vi "Update_FrontPanel.vi"(8 "End":timestamp, 9 "Start":timestamp, 11 "XYGraph in":refnum<vi>) -> ()   [LabVIEW 2020]
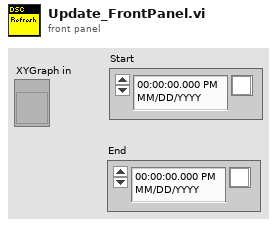
[diagram p1: front panel]
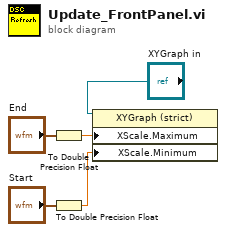
[diagram p0: block diagram]
diagram:
  n1 = To Double Precision Float(number="End") -> (double precision float=w3:dbl)
  n2 = To Double Precision Float(number="Start") -> (double precision float=w1:dbl)
  n3 = property on="Property Node" class="XYGraph (strict)"(reference="XYGraph in", "XScale.Maximum"=w3, "XScale.Minimum"=w1) -> ()  [unwired: 1 in, 2 out]
